vi "Simple_Example_dicam.vi"() -> ()   [LabVIEW 2019]
doc: "This example shows a simple recording of an image sequence with the pco.dicam C1,and the image access afterwards. It is a good starting point for writing own applications, but it will not be fail save, i.e. doesnt react on errors, just handles them forward to the end\nUsage:\nSelect your required image count and intensifier parameters before you start the program. Once started, the camera class will be initialized and images will be recorded automatically. When acquisition has finished you can address the images and crop them to a smaller size.To finish the program click on quit application, this will force fan exit of the camera class\nCaution: Overexposure to light can permanently damage the intensifier. Follow the precutions in the pco.dicam C1 manual to minimize the ridk of intensifier damage"
uses:
  camera/Camera.lvclass
  <vilib>/picture/picture.llb/Draw 8-Bit Pixmap.vi
  <vilib>/picture/picture.llb/Draw True-Color Pixmap.vi
  pco.sdk/SpecialCommandsDicam/SpecialCommandsDicam.lvlib
panel:
  out "strDescription":T1
  in  "delay_time":dbl=10.0 caption="delay time µs" max=4023.0
  in  "exp_time":dbl=10.0 caption="exp time µs" max=4023.0
  in  "loop_count":u32=10 caption="loop count" max=1
  in  "Intensified Gating":bool
  in  "MCP voltage":u32=1000 min=600 max=1000 step=10
  in  "decay_time":dbl=3033.0 caption="decay time" min=3033.0 max=10000.0 step=1.0
  out "colormap(U8)":u32[](array[numeric])
  out "Image(U16)":u16[][](graph)
  in  "Zoom [%]":i32(slide)=26 min=10 max=200 step=5 scale=10.0..200.0
  out "Image":picture
  out "rawImage":u16[][](array[numeric])
  in  "data_format":T2(ring)=enum."Mono16"
  in  "Image Index":u32 max=9
  out "Recorded Images":u32
  in  "Quit":bool
  in  "cropY1":u64=2 min=2 max=1504 step=1
  in  "cropX1":u64=2 min=2 max=1504 step=1
  in  "cropY0":u64=1 min=1 max=1503 step=1
  in  "cropX0":u64=1 min=1 max=1503 step=1
  out "Image Height":u16
  out "Image Width":u16
  in  "dwImgCount":u32=10 caption="Required Number of Images" max=4023
  out "Error":errorcluster {"code" format="%x"}
  # "This example shows a simple recording of an image sequence with the pco.dicam C1,and the image access afterwards.\nIt is a good starting point for writing own applications, but it will not be fail save, i.e. doesnt react on errors, just handles them forward to the end\nUsage:\nSelect your required image count  and intensifier parameters before you start the program. Once started, the camera class will be initialized and images will be recorded automatically. When acquisition has finished you can address the images and crop them to a smaller size.To finish the program click on quit application, this will force fan exit of the camera class\nCaution: Overexposure to light can permanently damage the intensifier. Follow the precutions in the pco.dicam C1 manual to minimize the ridk of intensifier damage"
  # "pco.labview"
  # "Dicam specific settings"
  # "Camera Setup"
  # "Recording Control"
  # "Parameters for image readout"
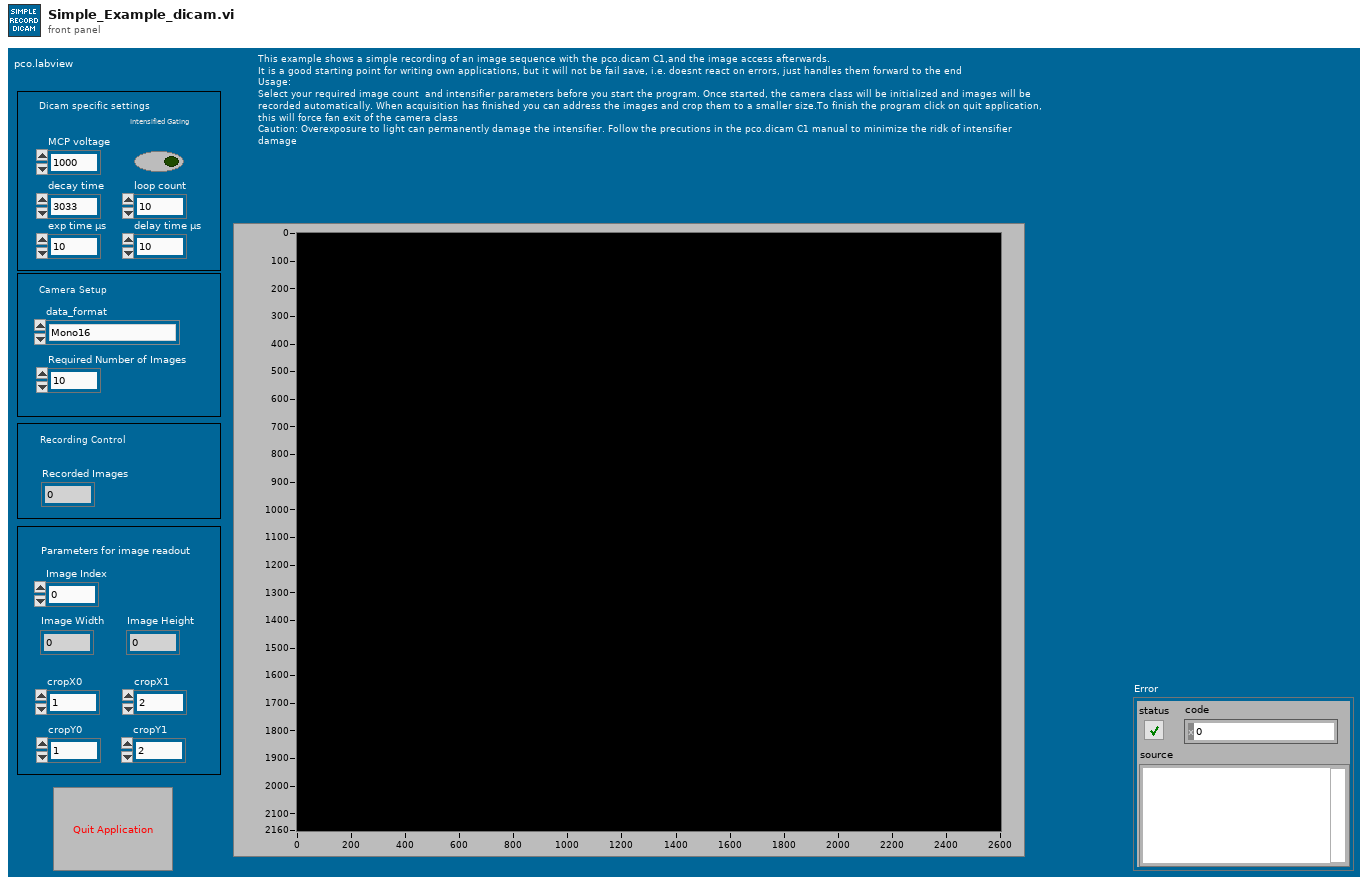
[diagram p1: front panel]
types:
  T1 = cluster{"wChannelNumberIntensifiedDESC":u16, "wNumberOfChannelsIntensifiedDESC":u16, "wMinVoltageIntensifiedDESC":u16, "wMaxVoltageIntensifiedDESC":u16, "wVoltageStepIntensifiedDESC":u16, "wExtendedMinVoltageIntensifiedDESC":u16, "wMaxLoopCountIntensifiedDESC":u16, "dwMinPhosphorDecayIntensified_ns_DESC":u32, "dwMaxPhosphorDecayIntensified_ms_DESC":u32, "dwFlagsIntensifiedDESC":u32, "szIntensifierTypeDESC":string, "dwMCP_RectangleXL_DESC":u32, "dwMCP_RectangleXR_DESC":u32, "dwMCP_RectangleYT_DESC":u32, "dwMCP_RectangleYB_DESC":u32}
  T2 = enum16{"Undefined", "Mono8", "Mono16", "BGRA8", "RGBA8", "BGRA16", "RGBA16", "CompressedMono8"}
  T3 = enum8{"Enabled", "Disabled", "Disabled and Grayed Out"}
  T4 = enum16{"sequence", "sequence non blocking", "ring buffer", "fifo", "tif", "multitif", "pcoraw", "b16", "dicom", "multidicom", "camram_ring", "camram_segment"}
  T5 = typedef "Camera.lvclass/binning.ctl" = cluster{"vert":u16, "horz":u16, "mode":u16}
  T6 = cluster{"exposure_time_s":dbl, "delay_time_s":dbl, "roi":cluster{"x0":u64, "y0":u64, "x1":u64, "y1":u64}, "timestamp_mode":u16, "pixelrate":u32, "conversion_factor":sgl, "trigger_mode":u16, "acquire_mode":u16, "acquire_sequence_number":u32, "metadata_mode":u16, "noisefilter_mode":u16, "pixel_format":u32, "binning":T5, "auto_exposure":cluster{"region":u16, "min_exposure_s":dbl, "max_exposure_s":dbl}}
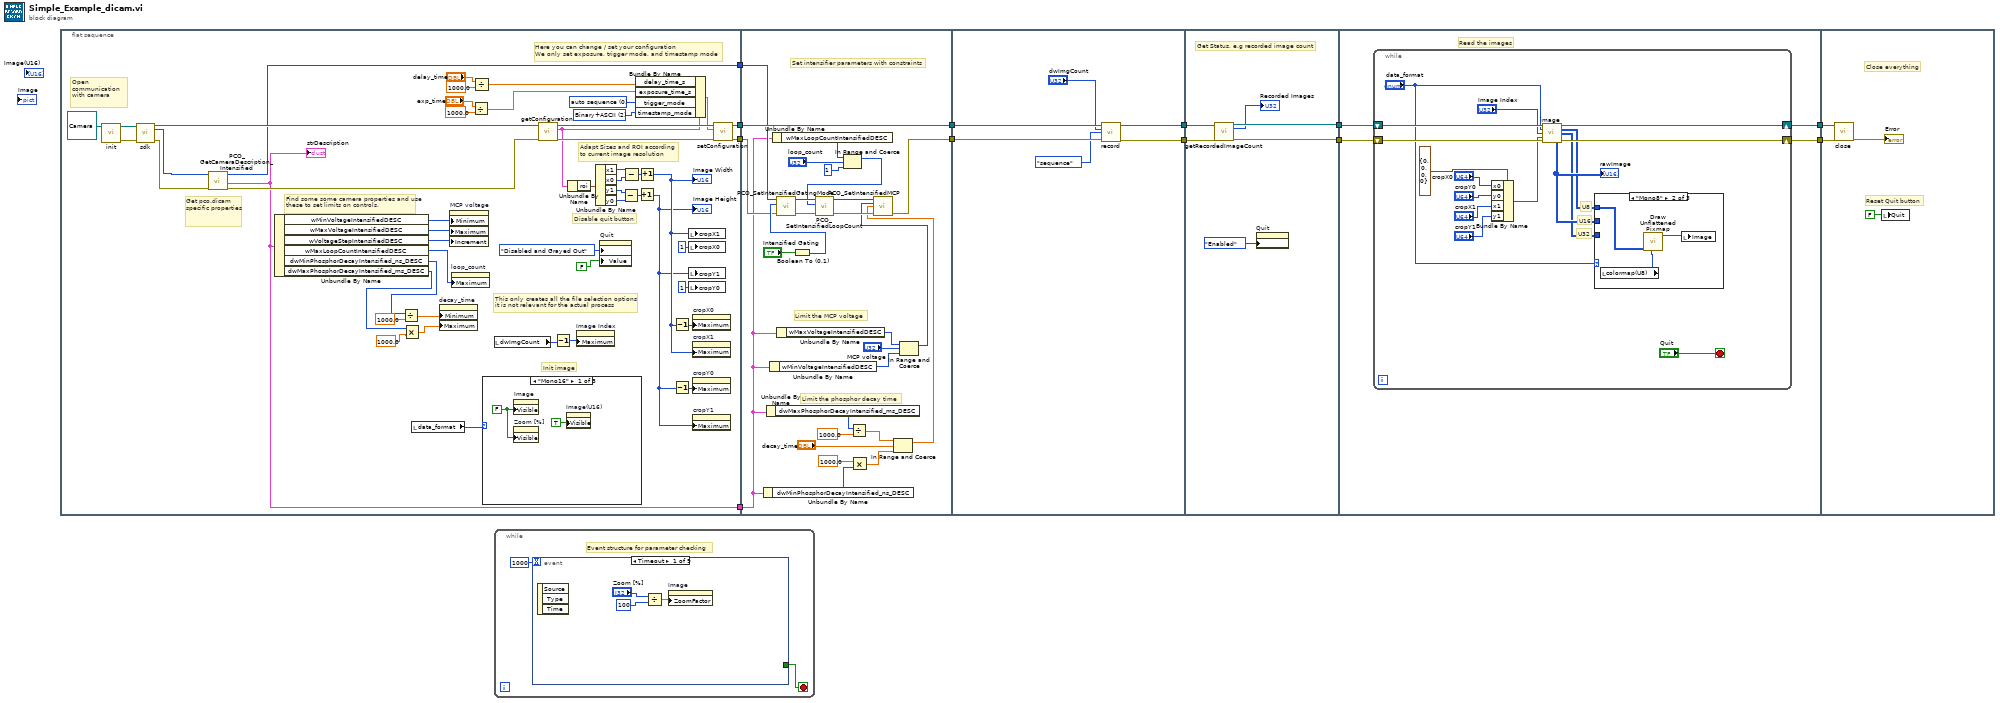
[diagram p0: block diagram]
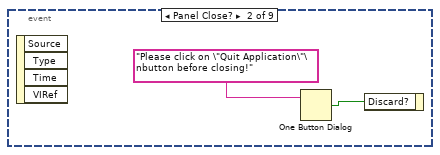
[diagram p2: hidden frame]
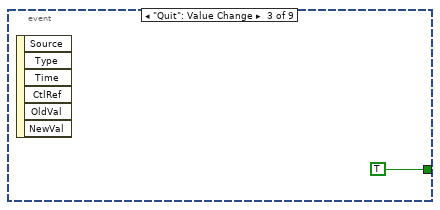
[diagram p3: hidden frame]
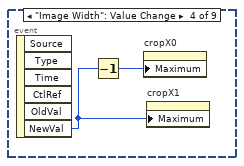
[diagram p4: hidden frame]
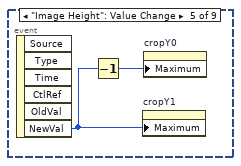
[diagram p5: hidden frame]
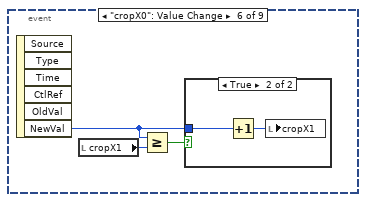
[diagram p6: hidden frame]
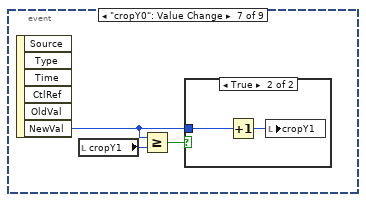
[diagram p8: hidden frame]
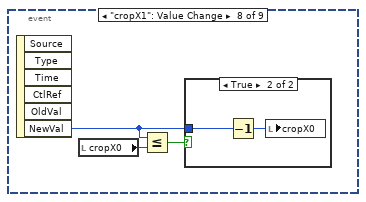
[diagram p10: hidden frame]
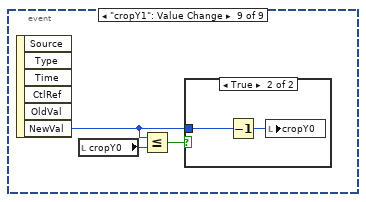
[diagram p12: hidden frame]
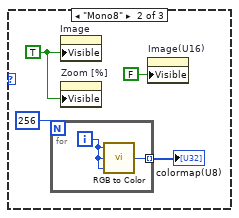
[diagram p14: hidden frame]
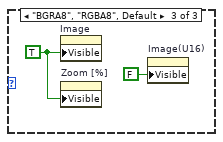
[diagram p15: hidden frame]
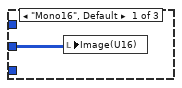
[diagram p16: hidden frame]
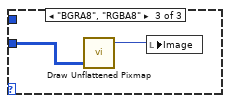
[diagram p17: hidden frame]
diagram:
  n1 = flat-sequence {
    tunnel: [w58] -> w6
    tunnel: [w57] -> w4
    tunnel: [w20] -> w2
    tunnel: [w13] -> w1
    tunnel: w6 -> [w100]
    tunnel: [w100] -> w5
    tunnel: w4 -> [w94]
    tunnel: [w91] -> w3
    tunnel: w2 -> [w99]
    tunnel: w1 -> [w80]
    tunnel: w5 -> [w106]
    tunnel: w3 -> [w105]
    tunnel: [w103] -> w12
    tunnel: [w102] -> w11
    tunnel: w12 -> [w112]
    tunnel: w11 -> [w111]
    tunnel: [w110] -> w10
    tunnel: [w109] -> w9
    tunnel: w10 -> [w115]
    tunnel: w9 -> [w116]
    tunnel: [w114] -> w8
    tunnel: [w113] -> w7
    tunnel: w8 -> [w140]
    tunnel: w7 -> [w139]
    frame #0 {
      w42 = u16 2 items=["OFF", "Binary", "Binary+ASCII", "ASCII"] ("TimestampMode")
      w62 = u16 0 items=["auto sequence"=0, "software trigger"=1, "external exposure start & software trigger"=2, "external exposure control"=3, "external synchronized"=4, "fast external exposure control"=5, "external CDS control"=6, "slow external exposure control"=7, "external synchronized HDSDI"=258] ("TriggerMode")
      # "Get pco.dicam specific properties"
      # "Find some some camera properties and use these to set limits on controls."
      # "Open communication with camera"
      # "Here you can change / set your configuration\nWe only set exposure, trigger mode, and timestamp mode"
      # "Init image"
      # "This only creates all the file selection options\nit is not relevant for the actual process"
      # "Adapt Sizes and ROI according\nto current image resolution"
      # "Disable quit button"
      n2 = call-dynamic "init.vi"("Camera in"=refnum<class "Camera.lvclass"> refnum ("PCOCamera in")) -> ("Camera out"=w36:refnum<class "Camera.lvclass">, "error out"=w35:errorcluster)  [unwired: 8 in]
      n3 = call-dynamic "sdk.vi"("Camera in"=w36, "error in (no error)"=w35) -> ("Camera out"=w34:refnum<class "Camera.lvclass">, "sdk"=w33:u64, "error out"=w32:errorcluster)  [unwired: 11 in]
      n4 = call "PCO_GetCameraDescription_Intensified.vi"("error in (no error)"=w32, "ph"=w33) -> ("error out"=w31:errorcluster, "strDescription"=w13:T1, "ph out"=w20:u64)  [unwired: 6 in, 1 out]
      "strDescription" <- w13
      n5 = Unbundle By Name(w13) -> ("wMinVoltageIntensifiedDESC"=w30:u16, "wMaxVoltageIntensifiedDESC"=w29:u16, "wVoltageStepIntensifiedDESC"=w28:u16, "wMaxLoopCountIntensifiedDESC"=w27:u16, "dwMinPhosphorDecayIntensified_ns_DESC"=w26:u32, "dwMaxPhosphorDecayIntensified_ms_DESC"=w23:u32)
      n6 = Divide(x=w26, y=1000.0) -> (x/y=w25:dbl)
      n7 = Multiply(x=w23, y=1000.0) -> (x*y=w21:dbl)
      n8 = local read "data_format"() -> (w37:T2)
      n9 = property on="decay_time" class="DigNum (strict)"("Minimum"=w25, "Maximum"=w21) -> ()  [unwired: 2 in, 2 out]
      n10 = property on="MCP voltage" class="DigNum (strict)"("Minimum"=w30, "Maximum"=w29, "Increment"=w28) -> ()  [unwired: 2 in, 2 out]
      n11 = property on="loop_count" class="DigNum (strict)"("Maximum"=w27) -> ()  [unwired: 2 in, 2 out]
      n12 = Divide(x="exp_time", y=1000.0) -> (x/y=w14:dbl)
      n13 = Divide(x="delay_time", y=1000.0) -> (x/y=w17:dbl)
      n14 = case shown="\"Mono16\"" w37 {
        frame "Mono16" {
          w65 = FALSE ("Visible")
          n15 = property on="Image" class="Pict"("Visible"=w65) -> ()  [unwired: 2 in, 2 out]
          n16 = property on="Zoom [%]" class="Slide (strict)"("Visible"=w65) -> ()  [unwired: 2 in, 2 out]
          n17 = property on="Image(U16)" class="IntGraph (strict)"("Visible"=TRUE) -> ()  [unwired: 2 in, 2 out]
        }
        frame "Mono8" {
          w68 = TRUE ("Visible")
          n18 = for {
            N: 256 -> [_]
            tunnel: [w70] -> w67 mode=indexing
            i -> [w71]
            n19 = call <vilib>:"RGB to Color.vi"("B"=w71, "G"=w71, "R"=w71) -> ("Color"=w70:u32)
          }
          "colormap(U8)" <- w67
          n20 = property on="Image" class="Pict"("Visible"=w68) -> ()  [unwired: 2 in, 2 out]
          n21 = property on="Zoom [%]" class="Slide (strict)"("Visible"=w68) -> ()  [unwired: 2 in, 2 out]
          n22 = property on="Image(U16)" class="IntGraph (strict)"("Visible"=FALSE) -> ()  [unwired: 2 in, 2 out]
        }
        frame "BGRA8", "RGBA8", Default {
          w72 = TRUE ("Visible")
          n23 = property on="Image" class="Pict"("Visible"=w72) -> ()  [unwired: 2 in, 2 out]
          n24 = property on="Zoom [%]" class="Slide (strict)"("Visible"=w72) -> ()  [unwired: 2 in, 2 out]
          n25 = property on="Image(U16)" class="IntGraph (strict)"("Visible"=FALSE) -> ()  [unwired: 2 in, 2 out]
        }
      }
      n26 = local read "dwImgCount"() -> (w38:u32)
      n27 = call-dynamic "getConfiguration.vi"("error in (no error)"=w31, "Camera in"=w34) -> ("error out"=w60:errorcluster, "configuration"=w52:T6, "Camera out"=w61:refnum<class "Camera.lvclass">)  [unwired: 7 in]
      n28 = Decrement(x=w38) -> (x-1=w39:u32)
      n29 = Unbundle By Name(w52) -> ("roi"=w51:cluster{"x0":u64, "y0":u64, "x1":u64, "y1":u64})
      n30 = property on="Image Index" class="DigNum (strict)"("Maximum"=w39) -> ()  [unwired: 2 in, 2 out]
      n31 = Unbundle By Name(w51) -> ("x1"=w49:u64, "x0"=w50:u64, "y1"=w47:u64, "y0"=w48:u64)
      n32 = property on="Quit" class="Bool (strict)"("DisabledEnum"=T3."Disabled and Grayed Out" ("Disabled"), "Value"=FALSE ("Stop")) -> ()  [unwired: 2 in, 2 out]
      n33 = Subtract(x=w47, y=w48) -> (x-y=w45:u64)
      n34 = Subtract(x=w49, y=w50) -> (x-y=w46:u64)
      n35 = Bundle By Name(cluster=w52, "delay_time_s"=w17, "exposure_time_s"=w14, "trigger_mode"=w62, "timestamp_mode"=w42) -> (w59:T6)
      n36 = Increment(x=w45) -> (x+1=w43:u64)
      "Image Height" <- w43
      n37 = Increment(x=w46) -> (x+1=w44:u64)
      "Image Width" <- w44
      n38 = Decrement(x=w44) -> (x-1=w54:u64)
      n39 = Decrement(x=w43) -> (x-1=w53:u64)
      n40 = local write "cropX1"(w44) -> ()
      n41 = local write "cropX0"(u16 1 ("roiY0")) -> ()
      n42 = local write "cropY1"(w43) -> ()
      n43 = local write "cropY0"(u16 1 ("roiY0")) -> ()
      n44 = property on="cropX0" class="DigNum (strict)"("Maximum"=w54) -> ()  [unwired: 2 in, 2 out]
      n45 = property on="cropX1" class="DigNum (strict)"("Maximum"=w44) -> ()  [unwired: 2 in, 2 out]
      n46 = property on="cropY0" class="DigNum (strict)"("Maximum"=w53) -> ()  [unwired: 2 in, 2 out]
      n47 = property on="cropY1" class="DigNum (strict)"("Maximum"=w43) -> ()  [unwired: 2 in, 2 out]
      n48 = call-dynamic "setConfiguration.vi"("error in (no error)"=w60, "configuration"=w59, "Camera in"=w61) -> ("error out"=w57:errorcluster, "Camera out"=w58:refnum<class "Camera.lvclass">)  [unwired: 7 in]
    }
    frame #1 {
      # "Limit the phosphor decay time"
      # "Limit the MCP voltage"
      # "Set intensifier parameters with constraints"
      n49 = Unbundle By Name(w80) -> ("dwMinPhosphorDecayIntensified_ns_DESC"=w78:u32)
      n50 = Unbundle By Name(w80) -> ("dwMaxPhosphorDecayIntensified_ms_DESC"=w82:u32)
      n51 = Unbundle By Name(w80) -> ("wMinVoltageIntensifiedDESC"=w84:u16)
      n52 = Unbundle By Name(w80) -> ("wMaxLoopCountIntensifiedDESC"=w90:u16)
      n53 = Unbundle By Name(w80) -> ("wMaxVoltageIntensifiedDESC"=w86:u16)
      n54 = Boolean To (0,1)(Boolean="Intensified Gating") -> (0, 1=w95:i16)
      n55 = call "PCO_SetIntensifiedGatingMode.vi"("error in (no error)"=w94, "wIntensifiedGatingMode"=w95, "ph"=w99) -> ("error out"=w97:errorcluster, "ph out"=w98:u64)  [unwired: 6 in, 1 out]
      n56 = In Range and Coerce(upper limit=w90, x="loop_count", lower limit=u32 1) -> (coerced(x)=w88:u32)  [unwired: 1 out]
      n57 = call "PCO_SetIntensifiedLoopCount.vi"("error in (no error)"=w97, "wIntensifiedLoopCount"=w88, "ph"=w98) -> ("error out"=w92:errorcluster, "ph out"=w93:u64)  [unwired: 6 in, 1 out]
      n58 = Divide(x=w82, y=1000.0) -> (x/y=w81:dbl)
      n59 = Multiply(x=1000.0, y=w78) -> (x*y=w77:dbl)
      n60 = In Range and Coerce(upper limit=w81, x="decay_time", lower limit=w77) -> (coerced(x)=w74:dbl)  [unwired: 1 out]
      n61 = In Range and Coerce(upper limit=w86, x="MCP voltage", lower limit=w84) -> (coerced(x)=w75:u32)  [unwired: 1 out]
      n62 = call "PCO_SetIntensifiedMCP.vi"("ph"=w93, "wIntensifiedVoltage"=w75, "dwIntensifiedPhosphorDecay_us"=w74, "error in (no error)"=w92) -> ("error out"=w91:errorcluster)  [unwired: 9 in, 2 out]
    }
    frame #2 {
      n63 = call-dynamic "record.vi"("Camera in"=w106, "num_images"="dwImgCount", "record_mode"=T4."sequence", "error in (no error)"=w105) -> ("Camera out"=w103:refnum<class "Camera.lvclass">, "error out"=w102:errorcluster)  [unwired: 10 in]
    }
    frame #3 {
      # "Get Status, e.g recorded image count"
      n64 = call-dynamic "getRecordedImageCount.vi"("Camera in"=w112, "error in (no error)"=w111) -> ("Camera out"=w110:refnum<class "Camera.lvclass">, "recorded_image_count"=→"Recorded Images":u32, "error out"=w109:errorcluster)  [unwired: 11 in]
      n65 = property on="Quit" class="Bool (strict)"("DisabledEnum"=T3."Enabled" ("Disabled")) -> ()  [unwired: 2 in, 2 out]
    }
    frame #4 {
      # "Read the images"
      n66 = while {
        shift-right: [w130] -> w114
        shift-left: w115 -> [w132]
        shift-right: [w125] -> w113
        shift-left: w116 -> [w131]
        stop <- "Quit" stop-if-true
        # "U32"
        # "U16"
        # "U8"
        n67 = Bundle By Name(cluster=cluster{"x0":u64, "y0":u64, "x1":u64, "y1":u64} {"x0"=0, "y0"=0, "x1"=0, "y1"=0} ("roi"), "x0"="cropX0", "y0"="cropY0", "x1"="cropX1", "y1"="cropY1") -> (w124:cluster{"x0":u64, "y0":u64, "x1":u64, "y1":u64})
        n68 = call-dynamic "image.vi"("Camera in"=w132, "data_format"="data_format", "image_index"="Image Index", "crop"=w124, "error in (no error)"=w131) -> ("Camera out"=w130:refnum<class "Camera.lvclass">, "image (U8)"=w117:u8[][], "image (U32)"=w118:u32[][], "raw_image (U16)"=w119:u16[][], "error out"=w125:errorcluster)  [unwired: 2 in, 4 out]
        "rawImage" <- w119
        n69 = case shown="\"Mono8\"" "data_format" {
          tunnel: w118 -> [_ _ w138]
          tunnel: w117 -> [_ w135 _]
          tunnel: w119 -> [w133 _ _]
          frame "Mono16", Default {
            n70 = local write "Image(U16)"(w133) -> ()
          }
          frame "Mono8" {
            n71 = local read "colormap(U8)"() -> (w134:u32[])
            n72 = call-poly <vilib>:"Draw Unflattened Pixmap.vi"("data"=w135, "color table"=w134) -> ("new picture"=w136:picture)  [unwired: 7 in]
            n73 = local write "Image"(w136) -> ()
          }
          frame "BGRA8", "RGBA8" {
            n74 = call-poly <vilib>:"Draw Unflattened Pixmap.vi"("data (RGB format)"=w138) -> ("new picture"=w137:picture)  [unwired: 8 in]
            n75 = local write "Image"(w137) -> ()
          }
        }
      }
    }
    frame #5 {
      # "Reset Quit button"
      # "Close everything"
      n76 = call-dynamic "close.vi"("error in (no error)"=w139, "Camera in"=w140) -> ("error out"=→"Error":errorcluster)  [unwired: 9 in]
      n77 = local write "Quit"(FALSE ("Stop")) -> ()
    }
  }
  n78 = while {
    stop <- w143 stop-if-true
    # "Event structure for parameter checking"
    n79 = event shown="[0] Timeout" {
      selector: _ -> [_ _ _ _ _ _ _ _ _]
      dyn-events: _ -> [_ _ _ _ _ _ _ _ _]
      timeout: 1000 -> [_ _ _ _ _ _ _ _ _]
      tunnel: [_ _ TRUE _ _ _ _ _ _] -> w143
      event Timeout {
        n80 = event-data() -> ()  [unwired: 1 in, 3 out]
        n81 = Divide(x="Zoom [%]", y=100 ("Zoom [%]")) -> (x/y=w145:dbl)
        n82 = property on="Image" class="Pict"("ZoomFactor"=w145) -> ()  [unwired: 2 in, 2 out]
      }
      event Panel Close? {
        n83 = event-data() -> ()  [unwired: 1 in, 4 out]
        n84 = One Button Dialog(message="Please click on \"Quit Application\"\nbutton before closing!") -> (true=w148:bool)  [unwired: 1 in]
        n85 = event-data("Discard?"=w148) -> ()  [unwired: 1 in, 1 out]
      }
      event "Quit": Value Change {
        n86 = event-data() -> ()  [unwired: 1 in, 6 out]
      }
      event "Image Width": Value Change {
        n87 = event-data() -> ("NewVal"=w151:u16)  [unwired: 1 in, 5 out]
        n88 = Decrement(x=w151) -> (x-1=w152:u16)
        n89 = property on="cropX0" class="DigNum (strict)"("Maximum"=w152) -> ()  [unwired: 2 in, 2 out]
        n90 = property on="cropX1" class="DigNum (strict)"("Maximum"=w151) -> ()  [unwired: 2 in, 2 out]
      }
      event "Image Height": Value Change {
        n91 = event-data() -> ("NewVal"=w153:u16)  [unwired: 1 in, 5 out]
        n92 = Decrement(x=w153) -> (x-1=w154:u16)
        n93 = property on="cropY1" class="DigNum (strict)"("Maximum"=w153) -> ()  [unwired: 2 in, 2 out]
        n94 = property on="cropY0" class="DigNum (strict)"("Maximum"=w154) -> ()  [unwired: 2 in, 2 out]
      }
      event "cropX0": Value Change {
        n95 = event-data() -> ("NewVal"=w155:u64)  [unwired: 1 in, 5 out]
        n96 = local read "cropX1"() -> (w157:u64)
        n97 = Greater Or Equal?(x=w155, y=w157) -> (x >= y?=w156:bool)
        n98 = case shown="True" w156 {
          tunnel: w155 -> [_ w159]
          frame False {
          }
          frame True {
            n99 = Increment(x=w159) -> (x+1=w158:u64)
            n100 = local write "cropX1"(w158) -> ()
          }
        }
      }
      event "cropY0": Value Change {
        n101 = event-data() -> ("NewVal"=w160:u64)  [unwired: 1 in, 5 out]
        n102 = local read "cropY1"() -> (w162:u64)
        n103 = Greater Or Equal?(x=w160, y=w162) -> (x >= y?=w161:bool)
        n104 = case shown="True" w161 {
          tunnel: w160 -> [_ w164]
          frame False {
          }
          frame True {
            n105 = Increment(x=w164) -> (x+1=w163:u64)
            n106 = local write "cropY1"(w163) -> ()
          }
        }
      }
      event "cropX1": Value Change {
        n107 = event-data() -> ("NewVal"=w165:u64)  [unwired: 1 in, 5 out]
        n108 = local read "cropX0"() -> (w167:u64)
        n109 = Less Or Equal?(x=w165, y=w167) -> (x <= y?=w166:bool)
        n110 = case shown="True" w166 {
          tunnel: w165 -> [_ w169]
          frame False {
          }
          frame True {
            n111 = Decrement(x=w169) -> (x-1=w168:u64)
            n112 = local write "cropX0"(w168) -> ()
          }
        }
      }
      event "cropY1": Value Change {
        n113 = event-data() -> ("NewVal"=w170:u64)  [unwired: 1 in, 5 out]
        n114 = local read "cropY0"() -> (w172:u64)
        n115 = Less Or Equal?(x=w170, y=w172) -> (x <= y?=w171:bool)
        n116 = case shown="True" w171 {
          tunnel: w170 -> [_ w174]
          frame False {
          }
          frame True {
            n117 = Decrement(x=w174) -> (x-1=w173:u64)
            n118 = local write "cropY0"(w173) -> ()
          }
        }
      }
    }
  }
